vi "使用ActiveX讀取Excel檔案 to XY Graph.vi"() -> ()   [LabVIEW 2016]
panel:
  out "XY Graph":cluster{dbl[], dbl[]}(graph) caption="XY Graph - dark"
  out "Sheets":string[][](table)=[["", "土壤濕度"], ["11/24/2022 11:00", "40.7"], ["11/24/2022 11:30", "36.4"], ["11/24/2022 12:00", "36.4"], ["11/24/2022 12:30", "38.9"], ["11/24/2022 13:00", "38.3"], ["11/24/2022 13:30", "37.7"], ["11/24/2022 14:00", "36.9"], ["11/24/2022 14:30", "36.2"], ["11/24/2022 15:00", "35.4"], ["11/24/2022 15:30", "34.6"], ["11/24/2022 16:00", "33.8"], ["11/24/2022 16:30", "33.3"], ["11/24/2022 17:00", "32.7"], ["11/24/2022 17:30", "31.9"], ["11/24/2022 18:00", "31.3"], ["11/24/2022 18:30", "31"], ["11/24/2022 19:00", "30.5"], ["11/24/2022 19:30", "30.1"], ["11/24/2022 20:00", "29.8"], ["11/24/2022 20:30", "29.6"], ["11/24/2022 21:00", "29.4"], ["11/24/2022 21:30", "29.2"], ["11/24/2022 22:00", "29.1"], ["11/24/2022 22:30", "28.9"], ["11/24/2022 23:00", "28.8"], ["11/24/2022 23:30", "28.6"], ["11/25/2022 00:00", "28.5"], ["11/25/2022 00:30", "28.3"], ["11/25/2022 01:00", "28.3"], ["11/25/2022 01:30", "28.1"], ["11/25/2022 02:00", "28.1"], ["11/25/2022 02:30", "27.9"], ["11/25/2022 03:00", "27.9"], ["11/25/2022 03:30", "27.7"], ["11/25/2022 04:00", "27.7"], ["11/25/2022 04:30", "27.6"], ["11/25/2022 05:00", "27.5"], ["11/25/2022 05:30", "27.4"], ["11/25/2022 06:00", "27.4"], ["11/25/2022 06:30", "27.3"], ["11/25/2022 07:00", "27.3"], ["11/25/2022 07:30", "27.1"], ["11/25/2022 08:00", "27.1"], ["11/25/2022 08:30", "27.1"], ["11/25/2022 09:00", "27.1"], ["11/25/2022 09:30", "27.1"], ["11/25/2022 10:00", "27"], ["11/25/2022 10:30", "26.9"], ["11/25/2022 11:00", "26.9"], ["11/25/2022 11:30", "26.7"], ["11/25/2022 12:00", "26.6"], ["11/25/2022 12:30", "26.4"], ["11/25/2022 13:00", "26.3"], ["11/25/2022 13:30", "26.2"], ["11/25/2022 14:00", "26.1"], ["11/25/2022 14:30", "26"], ["11/25/2022 15:00", "25.9"], ["11/25/2022 15:30", "25.8"], ["11/25/2022 16:00", "25.7"], ["11/25/2022 16:30", "25.7"], ["11/25/2022 17:00", "25.7"], ["11/25/2022 17:30", "25.5"], ["11/25/2022 18:00", "25.4"], ["11/25/2022 18:30", "25.4"], ["11/25/2022 19:00", "25.4"], ["11/25/2022 19:30", "25.4"], ["11/25/2022 20:00", "25.4"], ["11/25/2022 20:30", "25.4"], ["11/25/2022 21:00", "25.3"], ["11/25/2022 21:30", "25.3"], ["11/25/2022 22:00", "25.2"], ["11/25/2022 22:30", "25.2"], ["11/25/2022 23:00", "25.2"], ["11/25/2022 23:30", "25.2"], ["11/26/2022 00:00", "25.2"], ["11/26/2022 00:30", "25.2"], ["11/26/2022 01:00", "25.2"], ["11/26/2022 01:30", "25.2"], ["11/26/2022 02:00", "25.2"], ["11/26/2022 02:30", "25"], ["11/26/2022 03:00", "25"], ["11/26/2022 03:30", "25.1"], ["11/26/2022 04:00", "25"], ["11/26/2022 04:30", "25"], ["11/26/2022 05:00", "25.1"], ["11/26/2022 05:30", "25"], ["11/26/2022 06:00", "25"], ["11/26/2022 06:30", "25.1"], ["11/26/2022 07:00", "25"], ["11/26/2022 07:30", "24.9"], ["11/26/2022 08:00", "25"], ["11/26/2022 08:30", "25"], ["11/26/2022 09:00", "25"], ["11/26/2022 09:30", "26.5"], ["11/26/2022 10:00", "27.7"], ["11/26/2022 10:30", "28"], ["11/26/2022 11:00", "27.9"], ["11/26/2022 11:30", "27.8"], ["11/26/2022 12:00", "27.6"], ["11/26/2022 12:30", "27.4"], ["11/26/2022 13:00", "27.1"], ["11/26/2022 13:30", "27.1"], ["11/26/2022 14:00", "26.9"], ["11/26/2022 14:30", "26.7"], ["11/26/2022 15:00", "26.5"], ["11/26/2022 15:30", "26.3"], ["11/26/2022 16:00", "26.3"], ["11/26/2022 16:30", "26.1"], ["11/26/2022 17:00", "26"], ["11/26/2022 17:30", "26"], ["11/26/2022 18:00", "26"], ["11/26/2022 18:30", "25.9"], ["11/26/2022 19:00", "25.8"], ["11/26/2022 19:30", "25.7"], ["11/26/2022 20:00", "25.7"], ["11/26/2022 20:30", "25.6"], ["11/26/2022 21:00", "25.6"], ["11/26/2022 21:30", "25.5"], ["11/26/2022 22:00", "25.5"], ["11/26/2022 22:30", "25.4"], ["11/26/2022 23:00", "25.4"], ["11/26/2022 23:30", "25.4"], ["11/27/2022 00:00", "25.4"], ["11/27/2022 00:30", "25.4"], ["11/27/2022 01:00", "25.4"], ["11/27/2022 01:30", "25.3"], ["11/27/2022 02:00", "25.3"], ["11/27/2022 02:30", "25.2"], ["11/27/2022 03:00", "25.2"], ["11/27/2022 03:30", "25.2"], ["11/27/2022 04:00", "25.2"], ["11/27/2022 04:30", "25.2"], ["11/27/2022 05:00", "25.2"], ["11/27/2022 05:30", "25.1"], ["11/27/2022 06:00", "25.1"], ["11/27/2022 06:30", "25"], ["11/27/2022 07:00", "25.1"], ["11/27/2022 07:30", "25"], ["11/27/2022 08:00", "25"], ["11/27/2022 08:30", "25"], ["11/27/2022 09:00", "25"], ["11/27/2022 09:30", "25"], ["11/27/2022 10:00", "25"], ["11/27/2022 10:30", "25.1"], ["11/27/2022 11:00", "25.1"], ["11/27/2022 11:30", "25.1"], ["11/27/2022 12:00", "25.1"], ["11/27/2022 12:30", "25"], ["11/27/2022 13:00", "25"], ["11/27/2022 13:30", "25"], ["11/27/2022 14:00", "25"], ["11/27/2022 14:30", "25"], ["11/27/2022 15:00", "25"], ["11/27/2022 15:30", "25"], ["11/27/2022 16:00", "24.9"], ["11/27/2022 16:30", "24.9"], ["11/27/2022 17:00", "25"], ["11/27/2022 17:30", "24.9"], ["11/27/2022 18:00", "24.9"], ["11/27/2022 18:30", "24.8"], ["11/27/2022 19:00", "24.9"], ["11/27/2022 19:30", "24.8"], ["11/27/2022 20:00", "24.8"], ["11/27/2022 20:30", "24.8"], ["11/27/2022 21:00", "24.8"], ["11/27/2022 21:30", "24.8"], ["11/27/2022 22:00", "24.6"], ["11/27/2022 22:30", "24.8"], ["11/27/2022 23:00", "24.7"], ["11/27/2022 23:30", "24.7"], ["11/28/2022 00:00", "24.6"], ["11/28/2022 00:30", "24.6"], ["11/28/2022 01:00", "24.6"], ["11/28/2022 01:30", "24.6"], ["11/28/2022 02:00", "24.6"], ["11/28/2022 02:30", "24.6"], ["11/28/2022 03:00", "24.6"], ["11/28/2022 03:30", "24.5"], ["11/28/2022 04:00", "24.5"], ["11/28/2022 04:30", "24.5"], ["11/28/2022 05:00", "24.5"], ["11/28/2022 05:30", "24.5"], ["11/28/2022 06:00", "24.5"], ["11/28/2022 06:30", "24.4"], ["11/28/2022 07:00", "24.4"], ["11/28/2022 07:30", "24.4"], ["11/28/2022 08:00", "24.4"], ["11/28/2022 08:30", "24.5"], ["11/28/2022 09:00", "24.4"], ["11/28/2022 09:30", "24.5"], ["11/28/2022 10:00", "24.5"], ["11/28/2022 10:30", "24.6"], ["11/28/2022 11:00", "24.6"], ["11/28/2022 11:30", "24.6"], ["11/28/2022 12:00", "24.7"], ["11/28/2022 12:30", "24.6"], ["11/28/2022 13:00", "24.6"], ["11/28/2022 13:30", "24.7"], ["11/28/2022 14:00", "24.8"], ["11/28/2022 14:30", "24.7"], ["11/28/2022 15:00", "24.7"], ["11/28/2022 15:30", "24.7"], ["11/28/2022 16:00", "24.8"], ["11/28/2022 16:30", "24.7"], ["11/28/2022 17:00", "24.7"], ["11/28/2022 17:30", "24.6"], ["11/28/2022 18:00", "24.6"], ["11/28/2022 18:30", "24.5"], ["11/28/2022 19:00", "24.6"], ["11/28/2022 19:30", "24.6"], ["11/28/2022 20:00", "24.5"], ["11/28/2022 20:30", "24.5"], ["11/28/2022 21:00", "24.5"], ["11/28/2022 21:30", "24.5"], ["11/28/2022 22:00", "24.5"], ["11/28/2022 22:30", "24.3"], ["11/28/2022 23:00", "24.4"], ["11/28/2022 23:30", "24.4"], ["11/29/2022 00:00", "24.3"], ["11/29/2022 00:30", "24.3"], ["11/29/2022 01:00", "24.3"], ["11/29/2022 01:30", "24.3"], ["11/29/2022 02:00", "24.3"], ["11/29/2022 02:30", "24.3"], ["11/29/2022 03:00", "24.3"], ["11/29/2022 03:30", "24.3"], ["11/29/2022 04:00", "24.3"], ["11/29/2022 04:30", "24.3"], ["11/29/2022 05:00", "24.3"], ["11/29/2022 05:30", "24.2"], ["11/29/2022 06:00", "24.1"], ["11/29/2022 06:30", "24.2"], ["11/29/2022 07:00", "24.1"], ["11/29/2022 07:30", "24.2"], ["11/29/2022 08:00", "24.2"], ["11/29/2022 08:30", "24.1"], ["11/29/2022 09:00", "24.2"], ["11/29/2022 09:30", "24.1"], ["11/29/2022 10:00", "24.3"], ["11/29/2022 10:30", "24.3"], ["11/29/2022 11:00", "24.4"], ["11/29/2022 11:30", "24.4"], ["11/29/2022 12:00", "24.4"], ["11/29/2022 12:30", "24.5"], ["11/29/2022 13:00", "24.3"], ["11/29/2022 13:30", "24.5"], ["11/29/2022 14:00", "24.6"], ["11/29/2022 14:30", "24.6"], ["11/29/2022 15:00", "24.5"], ["11/29/2022 15:30", "24.5"], ["11/29/2022 16:00", "24.6"], ["11/29/2022 16:30", "24.6"], ["11/29/2022 17:00", "24.6"], ["11/29/2022 17:30", "24.6"], ["11/29/2022 18:00", "24.5"], ["11/29/2022 18:30", "24.5"], ["11/29/2022 19:00", "24.5"], ["11/29/2022 19:30", "24.4"], ["11/29/2022 20:00", "24.4"], ["11/29/2022 20:30", "24.5"], ["11/29/2022 21:00", "24.5"], ["11/29/2022 21:30", "24.4"], ["11/29/2022 22:00", "24.3"], ["11/29/2022 22:30", "24.3"], ["11/29/2022 23:00", "24.3"], ["11/29/2022 23:30", "24.3"], ["11/30/2022 00:00", "24.3"], ["11/30/2022 00:30", "24.3"], ["11/30/2022 01:00", "24.3"], ["11/30/2022 01:30", "24.3"], ["11/30/2022 02:00", "24.3"], ["11/30/2022 02:30", "24.2"], ["11/30/2022 03:00", "24.2"], ["11/30/2022 03:30", "24.2"], ["11/30/2022 04:00", "24.2"], ["11/30/2022 04:30", "24.1"], ["11/30/2022 05:00", "24.1"], ["11/30/2022 05:30", "24.1"], ["11/30/2022 06:00", "24.1"], ["11/30/2022 06:30", "24.1"], ["11/30/2022 07:00", "24.1"], ["11/30/2022 07:30", "24.1"], ["11/30/2022 08:00", "24.1"], ["11/30/2022 08:30", "24.1"], ["11/30/2022 09:00", "24.1"], ["11/30/2022 09:30", "24.1"], ["11/30/2022 10:00", "24.3"], ["11/30/2022 10:30", "24.3"], ["11/30/2022 11:00", "24.3"], ["11/30/2022 11:30", "24.3"], ["11/30/2022 12:00", "24.4"], ["11/30/2022 12:30", "24.3"], ["11/30/2022 13:00", "24.3"], ["11/30/2022 13:30", "24.3"], ["11/30/2022 14:00", "24.4"], ["11/30/2022 14:30", "24.4"], ["11/30/2022 15:00", "24.5"], ["11/30/2022 15:30", "24.4"], ["11/30/2022 16:00", "24.3"], ["11/30/2022 16:30", "24.4"], ["11/30/2022 17:00", "24.3"], ["11/30/2022 17:30", "24.3"], ["11/30/2022 18:00", "24.3"], ["11/30/2022 18:30", "24.3"], ["11/30/2022 19:00", "24.3"], ["11/30/2022 19:30", "24.2"], ["11/30/2022 20:00", "24.2"], ["11/30/2022 20:30", "24.1"], ["11/30/2022 21:00", "24.1"], ["11/30/2022 21:30", "24.2"], ["11/30/2022 22:00", "24.1"], ["11/30/2022 22:30", "24.1"], ["11/30/2022 23:00", "24.1"], ["11/30/2022 23:30", "24.1"], ["12/01/2022 00:00", "23.9"], ["12/01/2022 00:30", "24"], ["12/01/2022 01:00", "24.1"], ["12/01/2022 01:30", "24"], ["12/01/2022 02:00", "23.9"], ["12/01/2022 02:30", "23.9"], ["12/01/2022 03:00", "23.9"], ["12/01/2022 03:30", "23.9"], ["12/01/2022 04:00", "23.9"], ["12/01/2022 04:30", "23.9"], ["12/01/2022 05:00", "23.7"], ["12/01/2022 05:30", "23.8"], ["12/01/2022 06:00", "23.8"], ["12/01/2022 06:30", "23.7"], ["12/01/2022 07:00", "23.7"], ["12/01/2022 07:30", "23.7"], ["12/01/2022 08:00", "23.7"], ["12/01/2022 08:30", "23.7"], ["12/01/2022 09:00", "23.7"], ["12/01/2022 09:30", "23.9"], ["12/01/2022 10:00", "23.9"], ["12/01/2022 10:30", "24"], ["12/01/2022 11:00", "24"], ["12/01/2022 11:30", "24.1"], ["12/01/2022 12:00", "24.1"], ["12/01/2022 12:30", "24.1"], ["12/01/2022 13:00", "24.1"], ["12/01/2022 13:30", "24.1"], ["12/01/2022 14:00", "24.2"], ["12/01/2022 14:30", "24.1"], ["12/01/2022 15:00", "24.1"], ["12/01/2022 15:30", "24.2"], ["12/01/2022 16:00", "24.3"], ["12/01/2022 16:30", "24.2"], ["12/01/2022 17:00", "24.2"], ["12/01/2022 17:30", "24.1"], ["12/01/2022 18:00", "24.1"], ["12/01/2022 18:30", "24.1"], ["12/01/2022 19:00", "24.1"], ["12/01/2022 19:30", "24.1"], ["12/01/2022 20:00", "24.1"], ["12/01/2022 20:30", "24"], ["12/01/2022 21:00", "24.1"], ["12/01/2022 21:30", "24"], ["12/01/2022 22:00", "24"], ["12/01/2022 22:30", "23.9"], ["12/01/2022 23:00", "23.8"], ["12/01/2022 23:30", "23.8"], ["12/02/2022 00:00", "23.7"], ["12/02/2022 00:30", "23.8"], ["12/02/2022 01:00", "23.8"], ["12/02/2022 01:30", "23.7"], ["12/02/2022 02:00", "23.8"], ["12/02/2022 02:30", "23.8"], ["12/02/2022 03:00", "23.7"], ["12/02/2022 03:30", "23.7"], ["12/02/2022 04:00", "23.7"], ["12/02/2022 04:30", "23.7"], ["12/02/2022 05:00", "23.7"], ["12/02/2022 05:30", "23.7"], ["12/02/2022 06:00", "23.7"], ["12/02/2022 06:30", "23.7"], ["12/02/2022 07:00", "23.7"], ["12/02/2022 07:30", "23.7"], ["12/02/2022 08:00", "23.7"], ["12/02/2022 08:30", "23.7"], ["12/02/2022 09:00", "23.7"], ["12/02/2022 09:30", "24.1"], ["12/02/2022 10:00", "24.1"], ["12/02/2022 10:30", "24.1"], ["12/02/2022 11:00", "24.1"], ["12/02/2022 11:30", "24.1"], ["12/02/2022 12:00", "24.1"], ["12/02/2022 12:30", "24.1"], ["12/02/2022 13:00", "24.1"], ["12/02/2022 13:30", "24.1"], ["12/02/2022 14:00", "24.3"], ["12/02/2022 14:30", "24.3"], ["12/02/2022 15:00", "24.1"], ["12/02/2022 15:30", "24.1"], ["12/02/2022 16:00", "24.1"], ["12/02/2022 16:30", "24.2"], ["12/02/2022 17:00", "24.1"], ["12/02/2022 17:30", "23.8"], ["12/02/2022 18:00", "24.1"], ["12/02/2022 18:30", "24.1"], ["12/02/2022 19:00", "24.1"], ["12/02/2022 19:30", "24"], ["12/02/2022 20:00", "24.1"], ["12/02/2022 20:30", "23.9"], ["12/02/2022 21:00", "23.9"], ["12/02/2022 21:30", "23.9"], ["12/02/2022 22:00", "23.9"], ["12/02/2022 22:30", "23.9"], ["12/02/2022 23:00", "23.9"], ["12/02/2022 23:30", "23.7"], ["12/03/2022 00:00", "23.7"], ["12/03/2022 00:30", "23.8"], ["12/03/2022 01:00", "23.7"], ["12/03/2022 01:30", "23.7"], ["12/03/2022 02:00", "23.7"], ["12/03/2022 02:30", "23.7"], ["12/03/2022 03:00", "23.7"], ["12/03/2022 03:30", "23.6"], ["12/03/2022 04:00", "23.6"], ["12/03/2022 04:30", "23.5"], ["12/03/2022 05:00", "23.5"], ["12/03/2022 05:30", "23.5"], ["12/03/2022 06:00", "23.7"], ["12/03/2022 06:30", "23.6"], ["12/03/2022 07:00", "23.5"], ["12/03/2022 07:30", "23.5"], ["12/03/2022 08:00", "23.5"], ["12/03/2022 08:30", "23.5"], ["12/03/2022 09:00", "23.6"], ["12/03/2022 09:30", "23.7"], ["12/03/2022 10:00", "23.7"], ["12/03/2022 10:30", "23.8"], ["12/03/2022 11:00", "23.9"], ["12/03/2022 11:30", "23.9"], ["12/03/2022 12:00", "24"], ["12/03/2022 12:30", "24"], ["12/03/2022 13:00", "24"], ["12/03/2022 13:30", "23.9"], ["12/03/2022 14:00", "24.1"], ["12/03/2022 14:30", "24.1"], ["12/03/2022 15:00", "24.1"], ["12/03/2022 15:30", "24.1"], ["12/03/2022 16:00", "24.1"], ["12/03/2022 16:30", "24.1"], ["12/03/2022 17:00", "24.1"], ["12/03/2022 17:30", "24.1"], ["12/03/2022 18:00", "23.9"], ["12/03/2022 18:30", "24"], ["12/03/2022 19:00", "23.9"], ["12/03/2022 19:30", "23.9"], ["12/03/2022 20:00", "23.9"], ["12/03/2022 20:30", "23.9"], ["12/03/2022 21:00", "23.9"], ["12/03/2022 21:30", "23.7"], ["12/03/2022 22:00", "23.7"], ["12/03/2022 22:30", "23.7"], ["12/03/2022 23:00", "23.7"], ["12/03/2022 23:30", "23.7"], ["12/04/2022 00:00", "23.7"], ["12/04/2022 00:30", "23.7"], ["12/04/2022 01:00", "23.7"], ["12/04/2022 01:30", "23.7"], ["12/04/2022 02:00", "23.7"], ["12/04/2022 02:30", "23.7"], ["12/04/2022 03:00", "23.6"], ["12/04/2022 03:30", "23.5"], ["12/04/2022 04:00", "23.7"], ["12/04/2022 04:30", "23.6"], ["12/04/2022 05:00", "23.6"], ["12/04/2022 05:30", "23.6"], ["12/04/2022 06:00", "23.6"], ["12/04/2022 06:30", "23.6"], ["12/04/2022 07:00", "23.6"], ["12/04/2022 07:30", "23.5"], ["12/04/2022 08:00", "23.6"], ["12/04/2022 08:30", "23.5"], ["12/04/2022 09:00", "23.6"], ["12/04/2022 09:30", "23.7"], ["12/04/2022 10:00", "23.7"], ["12/04/2022 10:30", "23.7"], ["12/04/2022 11:00", "23.7"], ["12/04/2022 11:30", "23.7"], ["12/04/2022 12:00", "23.7"], ["12/04/2022 12:30", "23.8"], ["12/04/2022 13:00", "23.9"], ["12/04/2022 13:30", "23.9"], ["12/04/2022 14:00", "24"], ["12/04/2022 14:30", "23.9"], ["12/04/2022 15:00", "24.1"], ["12/04/2022 15:30", "24.1"], ["12/04/2022 16:00", "24.1"], ["12/04/2022 16:30", "24.1"], ["12/04/2022 17:00", "24.1"], ["12/04/2022 17:30", "23.9"], ["12/04/2022 18:00", "23.9"], ["12/04/2022 18:30", "23.9"], ["12/04/2022 19:00", "23.9"], ["12/04/2022 19:30", "23.7"], ["12/04/2022 20:00", "23.7"], ["12/04/2022 20:30", "23.7"], ["12/04/2022 21:00", "23.7"], ["12/04/2022 21:30", "23.7"], ["12/04/2022 22:00", "23.7"], ["12/04/2022 22:30", "23.7"], ["12/04/2022 23:00", "23.7"], ["12/04/2022 23:30", "23.7"], ["12/05/2022 00:00", "23.7"], ["12/05/2022 00:30", "23.7"], ["12/05/2022 01:00", "23.7"], ["12/05/2022 01:30", "23.7"], ["12/05/2022 02:00", "23.6"], ["12/05/2022 02:30", "23.5"], ["12/05/2022 03:00", "23.6"], ["12/05/2022 03:30", "23.6"], ["12/05/2022 04:00", "23.5"], ["12/05/2022 04:30", "23.5"], ["12/05/2022 05:00", "23.5"], ["12/05/2022 05:30", "23.5"], ["12/05/2022 06:00", "23.5"], ["12/05/2022 06:30", "23.5"], ["12/05/2022 07:00", "23.5"], ["12/05/2022 07:30", "23.5"], ["12/05/2022 08:00", "23.5"], ["12/05/2022 08:30", "23.5"], ["12/05/2022 09:00", "23.5"], ["12/05/2022 09:30", "23.6"], ["12/05/2022 10:00", "23.6"], ["12/05/2022 10:30", "23.7"], ["12/05/2022 11:00", "23.7"], ["12/05/2022 11:30", "23.9"], ["12/05/2022 12:00", "23.7"], ["12/05/2022 12:30", "23.7"], ["12/05/2022 13:00", "23.7"], ["12/05/2022 13:30", "23.9"], ["12/05/2022 14:00", "23.9"], ["12/05/2022 14:30", "23.8"], ["12/05/2022 15:00", "23.9"], ["12/05/2022 15:30", "23.8"], ["12/05/2022 16:00", "23.9"], ["12/05/2022 16:30", "23.9"], ["12/05/2022 17:00", "23.7"], ["12/05/2022 17:30", "23.8"], ["12/05/2022 18:00", "23.8"], ["12/05/2022 18:30", "23.7"], ["12/05/2022 19:00", "23.7"], ["12/05/2022 19:30", "23.7"], ["12/05/2022 20:00", "23.7"], ["12/05/2022 20:30", "23.6"], ["12/05/2022 21:00", "23.7"], ["12/05/2022 21:30", "23.5"], ["12/05/2022 22:00", "23.5"], ["12/05/2022 22:30", "23.5"], ["12/05/2022 23:00", "23.5"], ["12/05/2022 23:30", "23.5"], ["12/06/2022 00:00", "23.5"], ["12/06/2022 00:30", "23.5"], ["12/06/2022 01:00", "23.4"], ["12/06/2022 01:30", "23.5"], ["12/06/2022 02:00", "23.5"], ["12/06/2022 02:30", "23.5"], ["12/06/2022 03:00", "23.5"], ["12/06/2022 03:30", "23.4"], ["12/06/2022 04:00", "23.3"], ["12/06/2022 04:30", "23.4"], ["12/06/2022 05:00", "23.3"], ["12/06/2022 05:30", "23.3"], ["12/06/2022 06:00", "23.3"], ["12/06/2022 06:30", "23.3"], ["12/06/2022 07:00", "23.3"], ["12/06/2022 07:30", "23.3"], ["12/06/2022 08:00", "23.3"], ["12/06/2022 08:30", "23.3"], ["12/06/2022 09:00", "23.3"], ["12/06/2022 09:30", "23.3"], ["12/06/2022 10:00", "23.3"], ["12/06/2022 10:30", "23.4"], ["12/06/2022 11:00", "23.4"], ["12/06/2022 11:30", "23.5"], ["12/06/2022 12:00", "23.5"], ["12/06/2022 12:30", "23.5"], ["12/06/2022 13:00", "23.5"], ["12/06/2022 13:30", "23.6"], ["12/06/2022 14:00", "23.6"], ["12/06/2022 14:30", "23.6"], ["12/06/2022 15:00", "23.7"], ["12/06/2022 15:30", "23.7"], ["12/06/2022 16:00", "23.7"], ["12/06/2022 16:30", "23.5"], ["12/06/2022 17:00", "23.5"], ["12/06/2022 17:30", "23.4"], ["12/06/2022 18:00", "23.5"], ["12/06/2022 18:30", "23.5"], ["12/06/2022 19:00", "23.5"], ["12/06/2022 19:30", "23.4"], ["12/06/2022 20:00", "23.4"], ["12/06/2022 20:30", "23.3"], ["12/06/2022 21:00", "23.4"], ["12/06/2022 21:30", "23.3"], ["12/06/2022 22:00", "23.4"], ["12/06/2022 22:30", "23.3"], ["12/06/2022 23:00", "23.4"], ["12/06/2022 23:30", "23.3"], ["12/07/2022 00:00", "23.4"], ["12/07/2022 00:30", "23.3"], ["12/07/2022 01:00", "23.4"], ["12/07/2022 01:30", "23.3"], ["12/07/2022 02:00", "23.3"], ["12/07/2022 02:30", "23.3"], ["12/07/2022 03:00", "23.3"], ["12/07/2022 03:30", "23.3"], ["12/07/2022 04:00", "23.3"], ["12/07/2022 04:30", "23.3"], ["12/07/2022 05:00", "23.3"], ["12/07/2022 05:30", "23.3"], ["12/07/2022 06:00", "23.3"], ["12/07/2022 06:30", "23.3"], ["12/07/2022 07:00", "23.3"], ["12/07/2022 07:30", "23.3"], ["12/07/2022 08:00", "23.3"], ["12/07/2022 08:30", "23.3"], ["12/07/2022 09:00", "23.3"], ["12/07/2022 09:30", "23.3"], ["12/07/2022 10:00", "23.3"], ["12/07/2022 10:30", "23.5"], ["12/07/2022 11:00", "23.5"], ["12/07/2022 11:30", "23.5"], ["12/07/2022 12:00", "23.5"], ["12/07/2022 12:30", "23.5"], ["12/07/2022 13:00", "23.5"], ["12/07/2022 13:30", "23.5"], ["12/07/2022 14:00", "23.6"], ["12/07/2022 14:30", "23.5"], ["12/07/2022 15:00", "23.5"], ["12/07/2022 15:30", "23.5"], ["12/07/2022 16:00", "23.5"], ["12/07/2022 16:30", "23.5"], ["12/07/2022 17:00", "23.5"], ["12/07/2022 17:30", "23.5"], ["12/07/2022 18:00", "23.5"], ["12/07/2022 18:30", "23.5"], ["12/07/2022 19:00", "23.5"], ["12/07/2022 19:30", "23.5"], ["12/07/2022 20:00", "23.4"], ["12/07/2022 20:30", "23.4"], ["12/07/2022 21:00", "23.4"], ["12/07/2022 21:30", "23.3"], ["12/07/2022 22:00", "23.3"], ["12/07/2022 22:30", "23.4"], ["12/07/2022 23:00", "23.3"], ["12/07/2022 23:30", "23.3"], ["12/08/2022 00:00", "23.3"], ["12/08/2022 00:30", "23.3"], ["12/08/2022 01:00", "23.3"], ["12/08/2022 01:30", "23.2"], ["12/08/2022 02:00", "23.3"], ["12/08/2022 02:30", "23.2"], ["12/08/2022 03:00", "23.2"], ["12/08/2022 03:30", "23.1"], ["12/08/2022 04:00", "23.2"], ["12/08/2022 04:30", "23.2"], ["12/08/2022 05:00", "23.2"], ["12/08/2022 05:30", "23.2"], ["12/08/2022 06:00", "23.1"], ["12/08/2022 06:30", "23.2"], ["12/08/2022 07:00", "23.1"], ["12/08/2022 07:30", "23.1"], ["12/08/2022 08:00", "23"], ["12/08/2022 08:30", "23.1"], ["12/08/2022 09:00", "23"], ["12/08/2022 09:30", "23.1"], ["12/08/2022 10:00", "23.1"], ["12/08/2022 10:30", "23.2"], ["12/08/2022 11:00", "23.2"], ["12/08/2022 11:30", "23.3"], ["12/08/2022 12:00", "23.3"], ["12/08/2022 12:30", "23.4"], ["12/08/2022 13:00", "23.4"], ["12/08/2022 13:30", "23.4"], ["12/08/2022 14:00", "23.5"], ["12/08/2022 14:30", "23.5"], ["12/08/2022 15:00", "23.5"], ["12/08/2022 15:30", "23.5"], ["12/08/2022 16:00", "23.5"], ["12/08/2022 16:30", "23.3"], ["12/08/2022 17:00", "23.4"], ["12/08/2022 17:30", "23.5"], ["12/08/2022 18:00", "23.4"], ["12/08/2022 18:30", "23.5"], ["12/08/2022 19:00", "23.5"], ["12/08/2022 19:30", "23.5"], ["12/08/2022 20:00", "23.5"], ["12/08/2022 20:30", "23.4"], ["12/08/2022 21:00", "23.4"], ["12/08/2022 21:30", "23.3"], ["12/08/2022 22:00", "23.3"], ["12/08/2022 22:30", "23.3"], ["12/08/2022 23:00", "23.3"], ["12/08/2022 23:30", "23.2"], ["12/09/2022 00:00", "23.2"], ["12/09/2022 00:30", "23.2"], ["12/09/2022 01:00", "23.2"], ["12/09/2022 01:30", "23.2"], ["12/09/2022 02:00", "23.2"], ["12/09/2022 02:30", "23.2"], ["12/09/2022 03:00", "23.2"], ["12/09/2022 03:30", "23.1"], ["12/09/2022 04:00", "23"], ["12/09/2022 04:30", "23.1"], ["12/09/2022 05:00", "23"], ["12/09/2022 05:30", "23.1"], ["12/09/2022 06:00", "22.9"], ["12/09/2022 06:30", "22.9"], ["12/09/2022 07:00", "23"], ["12/09/2022 07:30", "23"], ["12/09/2022 08:00", "22.9"], ["12/09/2022 08:30", "22.9"], ["12/09/2022 09:00", "22.9"], ["12/09/2022 09:30", "22.8"], ["12/09/2022 10:00", "22.9"], ["12/09/2022 10:30", "22.9"], ["12/09/2022 11:00", "23.1"], ["12/09/2022 11:30", "23.2"], ["12/09/2022 12:00", "23.2"], ["12/09/2022 12:30", "23.1"], ["12/09/2022 13:00", "23.2"], ["12/09/2022 13:30", "23.3"], ["12/09/2022 14:00", "23.3"], ["12/09/2022 14:30", "23.3"], ["12/09/2022 15:00", "23.3"], ["12/09/2022 15:30", "23.3"], ["12/09/2022 16:00", "23.2"], ["12/09/2022 16:30", "23.3"], ["12/09/2022 17:00", "23.2"], ["12/09/2022 17:30", "23.2"], ["12/09/2022 18:00", "23.2"], ["12/09/2022 18:30", "23.2"], ["12/09/2022 19:00", "23.2"], ["12/09/2022 19:30", "23.2"], ["12/09/2022 20:00", "23.1"], ["12/09/2022 20:30", "23.1"], ["12/09/2022 21:00", "23.1"], ["12/09/2022 21:30", "23"], ["12/09/2022 22:00", "23.2"], ["12/09/2022 22:30", "23.2"], ["12/09/2022 23:00", "22.9"], ["12/09/2022 23:30", "23"], ["12/10/2022 00:00", "23.1"], ["12/10/2022 00:30", "23.1"], ["12/10/2022 01:00", "23"], ["12/10/2022 01:30", "22.9"], ["12/10/2022 02:00", "22.9"], ["12/10/2022 02:30", "22.9"], ["12/10/2022 03:00", "23.1"], ["12/10/2022 03:30", "22.9"], ["12/10/2022 04:00", "22.9"], ["12/10/2022 04:30", "22.9"], ["12/10/2022 05:00", "22.9"], ["12/10/2022 05:30", "22.9"], ["12/10/2022 06:00", "22.9"], ["12/10/2022 06:30", "22.9"], ["12/10/2022 07:00", "22.9"], ["12/10/2022 07:30", "22.9"], ["12/10/2022 08:00", "22.9"], ["12/10/2022 08:30", "22.9"], ["12/10/2022 09:00", "22.8"], ["12/10/2022 09:30", "22.9"], ["12/10/2022 10:00", "23.7"], ["12/10/2022 10:30", "24.3"], ["12/10/2022 11:00", "24.5"], ["12/10/2022 11:30", "24.6"], ["12/10/2022 12:00", "24.8"], ["12/10/2022 12:30", "24.8"], ["12/10/2022 13:00", "24.9"], ["12/10/2022 13:30", "24.9"], ["12/10/2022 14:00", "24.8"], ["12/10/2022 14:30", "24.8"], ["12/10/2022 15:00", "24.7"], ["12/10/2022 15:30", "24.7"], ["12/10/2022 16:00", "24.6"], ["12/10/2022 16:30", "24.6"], ["12/10/2022 17:00", "24.6"], ["12/10/2022 17:30", "24.5"], ["12/10/2022 18:00", "24.5"], ["12/10/2022 18:30", "24.5"], ["12/10/2022 19:00", "24.3"], ["12/10/2022 19:30", "24.4"], ["12/10/2022 20:00", "24.4"], ["12/10/2022 20:30", "24.3"], ["12/10/2022 21:00", "24.3"], ["12/10/2022 21:30", "24.3"], ["12/10/2022 22:00", "24.3"], ["12/10/2022 22:30", "24.2"], ["12/10/2022 23:00", "24.2"], ["12/10/2022 23:30", "24.2"], ["12/11/2022 00:00", "24.1"], ["12/11/2022 00:30", "24.1"], ["12/11/2022 01:00", "24"], ["12/11/2022 01:30", "24"], ["12/11/2022 02:00", "24"], ["12/11/2022 02:30", "24"], ["12/11/2022 03:00", "23.9"], ["12/11/2022 03:30", "23.8"], ["12/11/2022 04:00", "23.8"], ["12/11/2022 04:30", "23.7"], ["12/11/2022 05:00", "23.7"], ["12/11/2022 05:30", "23.7"], ["12/11/2022 06:00", "23.7"], ["12/11/2022 06:30", "23.7"], ["12/11/2022 07:00", "23.5"], ["12/11/2022 07:30", "23.6"], ["12/11/2022 08:00", "23.6"], ["12/11/2022 08:30", "23.5"], ["12/11/2022 09:00", "23.5"], ["12/11/2022 09:30", "23.5"], ["12/11/2022 10:00", "23.6"], ["12/11/2022 10:30", "23.5"], ["12/11/2022 11:00", "23.5"], ["12/11/2022 11:30", "23.6"], ["12/11/2022 12:00", "23.5"], ["12/11/2022 12:30", "23.5"], ["12/11/2022 13:00", "23.5"], ["12/11/2022 13:30", "23.5"], ["12/11/2022 14:00", "23.5"], ["12/11/2022 14:30", "23.5"], ["12/11/2022 15:00", "23.5"], ["12/11/2022 15:30", "23.5"], ["12/11/2022 16:00", "23.5"], ["12/11/2022 16:30", "23.5"], ["12/11/2022 17:00", "23.5"], ["12/11/2022 17:30", "23.5"], ["12/11/2022 18:00", "23.4"], ["12/11/2022 18:30", "23.5"], ["12/11/2022 19:00", "23.3"], ["12/11/2022 19:30", "23.5"], ["12/11/2022 20:00", "23.4"], ["12/11/2022 20:30", "23.3"], ["12/11/2022 21:00", "23.3"], ["12/11/2022 21:30", "23.4"], ["12/11/2022 22:00", "23.3"], ["12/11/2022 22:30", "23.3"], ["12/11/2022 23:00", "23.3"], ["12/11/2022 23:30", "23.2"], ["12/12/2022 00:00", "23.3"], ["12/12/2022 00:30", "23.3"], ["12/12/2022 01:00", "23.2"], ["12/12/2022 01:30", "23.2"], ["12/12/2022 02:00", "23.2"], ["12/12/2022 02:30", "23.1"], ["12/12/2022 03:00", "23.2"], ["12/12/2022 03:30", "23.1"], ["12/12/2022 04:00", "23.1"], ["12/12/2022 04:30", "23.1"], ["12/12/2022 05:00", "23.1"], ["12/12/2022 05:30", "23"], ["12/12/2022 06:00", "22.9"], ["12/12/2022 06:30", "23.1"], ["12/12/2022 07:00", "22.9"], ["12/12/2022 07:30", "22.9"], ["12/12/2022 08:00", "22.9"], ["12/12/2022 08:30", "22.9"], ["12/12/2022 09:00", "23"], ["12/12/2022 09:30", "22.9"], ["12/12/2022 10:00", "22.9"], ["12/12/2022 10:30", "22.9"], ["12/12/2022 11:00", "23.1"], ["12/12/2022 11:30", "23.1"], ["12/12/2022 12:00", "23.1"], ["12/12/2022 12:30", "23"], ["12/12/2022 13:00", "23.1"], ["12/12/2022 13:30", "23.1"], ["12/12/2022 14:00", "23.2"], ["12/12/2022 14:30", "23.1"], ["12/12/2022 15:00", "23.3"], ["12/12/2022 15:30", "23.2"], ["12/12/2022 16:00", "23.1"], ["12/12/2022 16:30", "23.1"], ["12/12/2022 17:00", "23.1"], ["12/12/2022 17:30", "23.1"], ["12/12/2022 18:00", "23"], ["12/12/2022 18:30", "22.9"], ["12/12/2022 19:00", "22.9"], ["12/12/2022 19:30", "23"], ["12/12/2022 20:00", "22.9"], ["12/12/2022 20:30", "22.9"], ["12/12/2022 21:00", "22.9"], ["12/12/2022 21:30", "22.9"], ["12/12/2022 22:00", "22.9"], ["12/12/2022 22:30", "22.9"], ["12/12/2022 23:00", "22.9"], ["12/12/2022 23:30", "22.9"], ["12/13/2022 00:00", "22.9"], ["12/13/2022 00:30", "22.9"], ["12/13/2022 01:00", "22.8"], ["12/13/2022 01:30", "22.9"], ["12/13/2022 02:00", "22.8"], ["12/13/2022 02:30", "22.8"], ["12/13/2022 03:00", "22.8"], ["12/13/2022 03:30", "22.7"], ["12/13/2022 04:00", "22.7"], ["12/13/2022 04:30", "22.8"], ["12/13/2022 05:00", "22.7"], ["12/13/2022 05:30", "22.7"], ["12/13/2022 06:00", "22.7"], ["12/13/2022 06:30", "22.7"], ["12/13/2022 07:00", "22.7"], ["12/13/2022 07:30", "22.7"], ["12/13/2022 08:00", "22.7"], ["12/13/2022 08:30", "22.7"], ["12/13/2022 09:00", "22.7"], ["12/13/2022 09:30", "22.7"], ["12/13/2022 10:00", "22.8"], ["12/13/2022 10:30", "22.8"], ["12/13/2022 11:00", "22.9"], ["12/13/2022 11:30", "22.9"], ["12/13/2022 12:00", "22.9"], ["12/13/2022 12:30", "22.9"], ["12/13/2022 13:00", "22.9"], ["12/13/2022 13:30", "22.9"], ["12/13/2022 14:00", "22.9"], ["12/13/2022 14:30", "23.1"], ["12/13/2022 15:00", "23.1"], ["12/13/2022 15:30", "23.1"], ["12/13/2022 16:00", "23"], ["12/13/2022 16:30", "23.1"], ["12/13/2022 17:00", "22.9"], ["12/13/2022 17:30", "22.9"], ["12/13/2022 18:00", "23.1"], ["12/13/2022 18:30", "23.1"], ["12/13/2022 19:00", "22.9"], ["12/13/2022 19:30", "22.9"], ["12/13/2022 20:00", "22.9"], ["12/13/2022 20:30", "22.8"], ["12/13/2022 21:00", "22.9"], ["12/13/2022 21:30", "22.8"], ["12/13/2022 22:00", "22.8"], ["12/13/2022 22:30", "22.8"], ["12/13/2022 23:00", "22.8"], ["12/13/2022 23:30", "22.7"], ["12/14/2022 00:00", "22.7"], ["12/14/2022 00:30", "22.7"], ["12/14/2022 01:00", "22.7"], ["12/14/2022 01:30", "22.7"], ["12/14/2022 02:00", "22.7"], ["12/14/2022 02:30", "22.7"], ["12/14/2022 03:00", "22.7"], ["12/14/2022 03:30", "22.7"], ["12/14/2022 04:00", "22.7"], ["12/14/2022 04:30", "22.7"], ["12/14/2022 05:00", "22.7"], ["12/14/2022 05:30", "22.6"], ["12/14/2022 06:00", "22.6"], ["12/14/2022 06:30", "22.6"], ["12/14/2022 07:00", "22.6"], ["12/14/2022 07:30", "22.7"], ["12/14/2022 08:00", "22.6"], ["12/14/2022 08:30", "22.5"], ["12/14/2022 09:00", "22.6"], ["12/14/2022 09:30", "22.7"], ["12/14/2022 10:00", "22.5"], ["12/14/2022 10:30", "22.7"], ["12/14/2022 11:00", "22.7"], ["12/14/2022 11:30", "22.7"], ["12/14/2022 12:00", "22.7"], ["12/14/2022 12:30", "22.7"], ["12/14/2022 13:00", "22.7"], ["12/14/2022 13:30", "22.7"], ["12/14/2022 14:00", "22.7"], ["12/14/2022 14:30", "22.8"], ["12/14/2022 15:00", "22.8"], ["12/14/2022 15:30", "22.7"], ["12/14/2022 16:00", "22.7"], ["12/14/2022 16:30", "22.7"], ["12/14/2022 17:00", "22.7"], ["12/14/2022 17:30", "22.8"], ["12/14/2022 18:00", "22.8"], ["12/14/2022 18:30", "22.7"], ["12/14/2022 19:00", "22.7"], ["12/14/2022 19:30", "22.8"], ["12/14/2022 20:00", "22.7"], ["12/14/2022 20:30", "22.7"], ["12/14/2022 21:00", "22.7"], ["12/14/2022 21:30", "22.7"], ["12/14/2022 22:00", "22.7"], ["12/14/2022 22:30", "22.7"], ["12/14/2022 23:00", "22.7"], ["12/14/2022 23:30", "22.7"], ["12/15/2022 00:00", "22.7"], ["12/15/2022 00:30", "22.6"], ["12/15/2022 01:00", "22.7"], ["12/15/2022 01:30", "22.7"], ["12/15/2022 02:00", "22.7"], ["12/15/2022 02:30", "22.6"], ["12/15/2022 03:00", "22.6"], ["12/15/2022 03:30", "22.7"], ["12/15/2022 04:00", "22.6"], ["12/15/2022 04:30", "22.6"], ["12/15/2022 05:00", "22.5"], ["12/15/2022 05:30", "22.6"], ["12/15/2022 06:00", "22.6"], ["12/15/2022 06:30", "22.6"], ["12/15/2022 07:00", "22.6"], ["12/15/2022 07:30", "22.6"], ["12/15/2022 08:00", "22.5"], ["12/15/2022 08:30", "22.6"], ["12/15/2022 09:00", "22.5"], ["12/15/2022 09:30", "22.5"], ["12/15/2022 10:00", "22.7"], ["12/15/2022 10:30", "22.7"], ["12/15/2022 11:00", "22.7"], ["12/15/2022 11:30", "22.7"], ["12/15/2022 12:00", "22.8"], ["12/15/2022 12:30", "22.8"], ["12/15/2022 13:00", "22.7"], ["12/15/2022 13:30", "22.9"], ["12/15/2022 14:00", "22.8"], ["12/15/2022 14:30", "22.9"], ["12/15/2022 15:00", "22.9"], ["12/15/2022 15:30", "22.8"], ["12/15/2022 16:00", "22.9"], ["12/15/2022 16:30", "22.9"], ["12/15/2022 17:00", "22.9"], ["12/15/2022 17:30", "22.7"], ["12/15/2022 18:00", "22.9"], ["12/15/2022 18:30", "22.9"], ["12/15/2022 19:00", "22.8"], ["12/15/2022 19:30", "22.8"], ["12/15/2022 20:00", "22.9"], ["12/15/2022 20:30", "22.8"], ["12/15/2022 21:00", "22.7"], ["12/15/2022 21:30", "22.7"], ["12/15/2022 22:00", "22.8"], ["12/15/2022 22:30", "22.7"], ["12/15/2022 23:00", "22.8"], ["12/15/2022 23:30", "22.7"], ["12/16/2022 00:00", "22.7"], ["12/16/2022 00:30", "22.7"], ["12/16/2022 01:00", "22.8"], ["12/16/2022 01:30", "22.7"], ["12/16/2022 02:00", "22.7"], ["12/16/2022 02:30", "22.7"], ["12/16/2022 03:00", "22.6"], ["12/16/2022 03:30", "22.7"], ["12/16/2022 04:00", "22.7"], ["12/16/2022 04:30", "22.7"], ["12/16/2022 05:00", "22.7"], ["12/16/2022 05:30", "22.7"], ["12/16/2022 06:00", "22.7"], ["12/16/2022 06:30", "22.6"], ["12/16/2022 07:00", "22.6"], ["12/16/2022 07:30", "22.6"], ["12/16/2022 08:00", "22.7"], ["12/16/2022 08:30", "22.6"], ["12/16/2022 09:00", "22.7"], ["12/16/2022 09:30", "22.6"], ["12/16/2022 10:00", "22.7"], ["12/16/2022 10:30", "22.8"], ["12/16/2022 11:00", "22.8"], ["12/16/2022 11:30", "22.7"], ["12/16/2022 12:00", "22.8"], ["12/16/2022 12:30", "22.9"], ["12/16/2022 13:00", "22.9"], ["12/16/2022 13:30", "22.9"], ["12/16/2022 14:00", "22.9"], ["12/16/2022 14:30", "22.9"], ["12/16/2022 15:00", "22.9"], ["12/16/2022 15:30", "22.9"], ["12/16/2022 16:00", "22.9"], ["12/16/2022 16:30", "22.9"], ["12/16/2022 17:00", "22.9"], ["12/16/2022 17:30", "22.8"], ["12/16/2022 18:00", "22.9"], ["12/16/2022 18:30", "22.8"], ["12/16/2022 19:00", "22.8"], ["12/16/2022 19:30", "22.8"], ["12/16/2022 20:00", "22.8"], ["12/16/2022 20:30", "22.7"], ["12/16/2022 21:00", "22.7"], ["12/16/2022 21:30", "22.7"], ["12/16/2022 22:00", "22.7"], ["12/16/2022 22:30", "22.7"], ["12/16/2022 23:00", "22.7"], ["12/16/2022 23:30", "22.7"], ["12/17/2022 00:00", "22.7"], ["12/17/2022 00:30", "22.7"], ["12/17/2022 01:00", "22.7"], ["12/17/2022 01:30", "22.7"], ["12/17/2022 02:00", "22.7"], ["12/17/2022 02:30", "22.7"], ["12/17/2022 03:00", "22.7"], ["12/17/2022 03:30", "22.5"], ["12/17/2022 04:00", "22.5"], ["12/17/2022 04:30", "22.6"], ["12/17/2022 05:00", "22.6"], ["12/17/2022 05:30", "22.7"], ["12/17/2022 06:00", "22.6"], ["12/17/2022 06:30", "22.4"], ["12/17/2022 07:00", "22.5"], ["12/17/2022 07:30", "22.4"], ["12/17/2022 08:00", "22.4"], ["12/17/2022 08:30", "22.4"], ["12/17/2022 09:00", "22.4"], ["12/17/2022 09:30", "22.4"], ["12/17/2022 10:00", "22.7"], ["12/17/2022 10:30", "22.7"], ["12/17/2022 11:00", "22.6"], ["12/17/2022 11:30", "22.5"], ["12/17/2022 12:00", "22.6"], ["12/17/2022 12:30", "22.5"], ["12/17/2022 13:00", "22.9"], ["12/17/2022 13:30", "22.9"], ["12/17/2022 14:00", "23.1"], ["12/17/2022 14:30", "23.2"], ["12/17/2022 15:00", "23.2"], ["12/17/2022 15:30", "23.2"], ["12/17/2022 16:00", "23.3"], ["12/17/2022 16:30", "23.3"], ["12/17/2022 17:00", "23.4"], ["12/17/2022 17:30", "23.3"], ["12/17/2022 18:00", "23.4"], ["12/17/2022 18:30", "23.4"], ["12/17/2022 19:00", "23.4"], ["12/17/2022 19:30", "23.3"], ["12/17/2022 20:00", "23.5"], ["12/17/2022 20:30", "23.5"], ["12/17/2022 21:00", "23.3"], ["12/17/2022 21:30", "23.4"], ["12/17/2022 22:00", "23.3"], ["12/17/2022 22:30", "23.1"], ["12/17/2022 23:00", "23.3"], ["12/17/2022 23:30", "23.4"], ["12/18/2022 00:00", "23.5"], ["12/18/2022 00:30", "23.5"], ["12/18/2022 01:00", "23.4"], ["12/18/2022 01:30", "23.5"], ["12/18/2022 02:00", "23.6"], ["12/18/2022 02:30", "23.8"], ["12/18/2022 03:00", "23.9"], ["12/18/2022 03:30", "24.1"], ["12/18/2022 04:00", "24"], ["12/18/2022 04:30", "24.1"], ["12/18/2022 05:00", "24.1"], ["12/18/2022 05:30", "24.1"], ["12/18/2022 06:00", "24"], ["12/18/2022 06:30", "24.1"], ["12/18/2022 07:00", "24.1"], ["12/18/2022 07:30", "24.1"], ["12/18/2022 08:00", "24"], ["12/18/2022 08:30", "23.9"], ["12/18/2022 09:00", "23.9"], ["12/18/2022 09:30", "23.9"], ["12/18/2022 10:00", "24"], ["12/18/2022 10:30", "24"], ["12/18/2022 11:00", "23.9"], ["12/18/2022 11:30", "24"], ["12/18/2022 12:00", "24"], ["12/18/2022 12:30", "24"], ["12/18/2022 13:00", "24"], ["12/18/2022 13:30", "24"], ["12/18/2022 14:00", "24"], ["12/18/2022 14:30", "23.9"], ["12/18/2022 15:00", "23.9"], ["12/18/2022 15:30", "23.9"], ["12/18/2022 16:00", "24"], ["12/18/2022 16:30", "23.9"], ["12/18/2022 17:00", "23.9"], ["12/18/2022 17:30", "23.7"], ["12/18/2022 18:00", "23.7"], ["12/18/2022 18:30", "23.7"], ["12/18/2022 19:00", "23.7"], ["12/18/2022 19:30", "23.7"], ["12/18/2022 20:00", "23.7"], ["12/18/2022 20:30", "23.7"], ["12/18/2022 21:00", "23.7"], ["12/18/2022 21:30", "23.7"], ["12/18/2022 22:00", "23.5"], ["12/18/2022 22:30", "23.6"], ["12/18/2022 23:00", "23.5"], ["12/18/2022 23:30", "23.5"], ["12/19/2022 00:00", "23.5"], ["12/19/2022 00:30", "23.6"], ["12/19/2022 01:00", "23.5"], ["12/19/2022 01:30", "23.5"], ["12/19/2022 02:00", "23.5"], ["12/19/2022 02:30", "23.5"], ["12/19/2022 03:00", "23.5"], ["12/19/2022 03:30", "23.5"], ["12/19/2022 04:00", "23.5"], ["12/19/2022 04:30", "23.4"], ["12/19/2022 05:00", "23.4"], ["12/19/2022 05:30", "23.3"], ["12/19/2022 06:00", "23.4"], ["12/19/2022 06:30", "23.4"], ["12/19/2022 07:00", "23.3"], ["12/19/2022 07:30", "23.3"], ["12/19/2022 08:00", "23.3"], ["12/19/2022 08:30", "23.3"], ["12/19/2022 09:00", "23.5"], ["12/19/2022 09:30", "23.5"], ["12/19/2022 10:00", "23.5"], ["12/19/2022 10:30", "23.5"], ["12/19/2022 11:00", "23.5"], ["12/19/2022 11:30", "23.5"], ["12/19/2022 12:00", "23.5"], ["12/19/2022 12:30", "23.5"], ["12/19/2022 13:00", "23.5"], ["12/19/2022 13:30", "23.5"], ["12/19/2022 14:00", "23.5"], ["12/19/2022 14:30", "23.6"], ["12/19/2022 15:00", "23.6"], ["12/19/2022 15:30", "23.5"], ["12/19/2022 16:00", "23.5"], ["12/19/2022 16:30", "23.6"], ["12/19/2022 17:00", "23.6"], ["12/19/2022 17:30", "23.5"], ["12/19/2022 18:00", "23.6"], ["12/19/2022 18:30", "23.5"], ["12/19/2022 19:00", "23.5"], ["12/19/2022 19:30", "23.5"], ["12/19/2022 20:00", "23.4"], ["12/19/2022 20:30", "23.4"], ["12/19/2022 21:00", "23.3"], ["12/19/2022 21:30", "23.4"], ["12/19/2022 22:00", "23.3"], ["12/19/2022 22:30", "23.3"], ["12/19/2022 23:00", "23.3"], ["12/19/2022 23:30", "23.2"], ["12/20/2022 00:00", "23.2"], ["12/20/2022 00:30", "23.1"], ["12/20/2022 01:00", "23.2"], ["12/20/2022 01:30", "23.2"], ["12/20/2022 02:00", "22.9"], ["12/20/2022 02:30", "23.1"], ["12/20/2022 03:00", "23"], ["12/20/2022 03:30", "23.1"], ["12/20/2022 04:00", "22.9"], ["12/20/2022 04:30", "23"], ["12/20/2022 05:00", "22.9"], ["12/20/2022 05:30", "22.9"], ["12/20/2022 06:00", "22.9"], ["12/20/2022 06:30", "22.9"], ["12/20/2022 07:00", "22.9"], ["12/20/2022 07:30", "22.8"], ["12/20/2022 08:00", "22.8"], ["12/20/2022 08:30", "22.9"], ["12/20/2022 09:00", "22.9"], ["12/20/2022 09:30", "22.9"], ["12/20/2022 10:00", "23.7"], ["12/20/2022 10:30", "27.1"], ["12/20/2022 11:00", "28.6"], ["12/20/2022 11:30", "29.8"], ["12/20/2022 12:00", "31.3"], ["12/20/2022 12:30", "31.8"], ["12/20/2022 13:00", "32"], ["12/20/2022 13:30", "32.1"], ["12/20/2022 14:00", "32.1"], ["12/20/2022 14:30", "32.1"], ["12/20/2022 15:00", "32"], ["12/20/2022 15:30", "31.8"], ["12/20/2022 16:00", "31.6"], ["12/20/2022 16:30", "31.3"], ["12/20/2022 17:00", "31.1"]]
  in  "範圍":cluster{"Cell1":string, "Cell2":string}={"Cell1"="A1", "Cell2"="B1262"}
  in  "Sheets":i32=1
  in  "Path":path
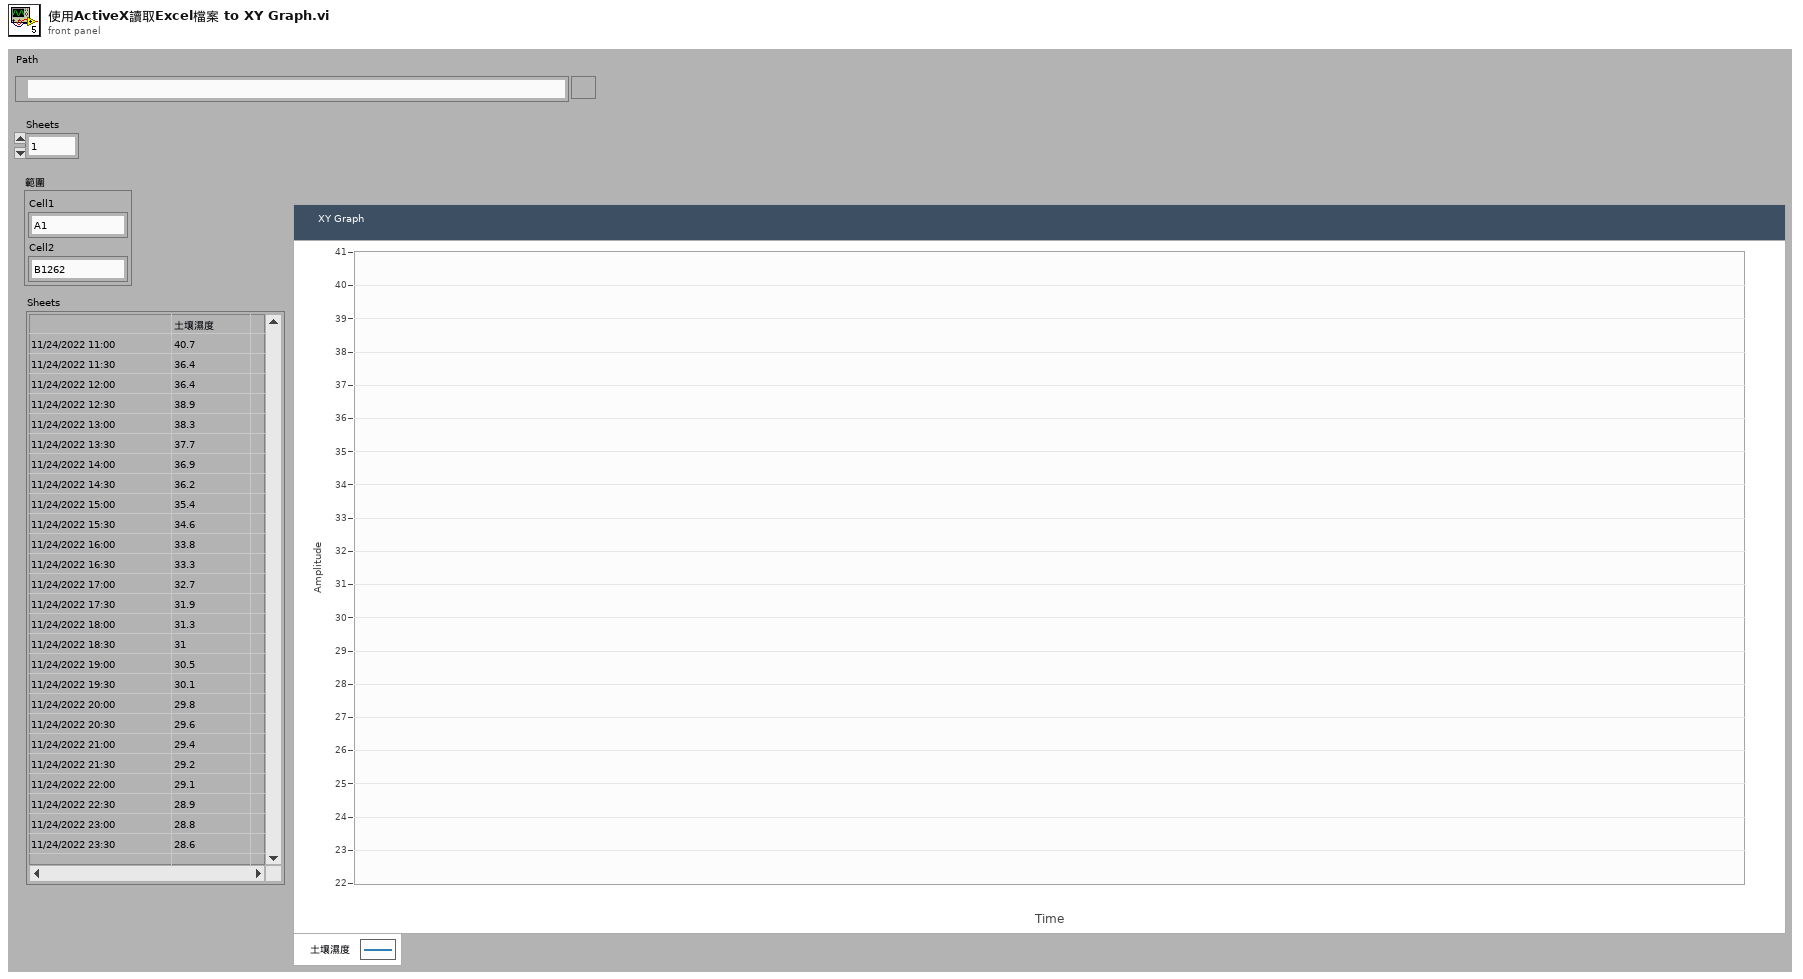
[diagram p1: front panel]
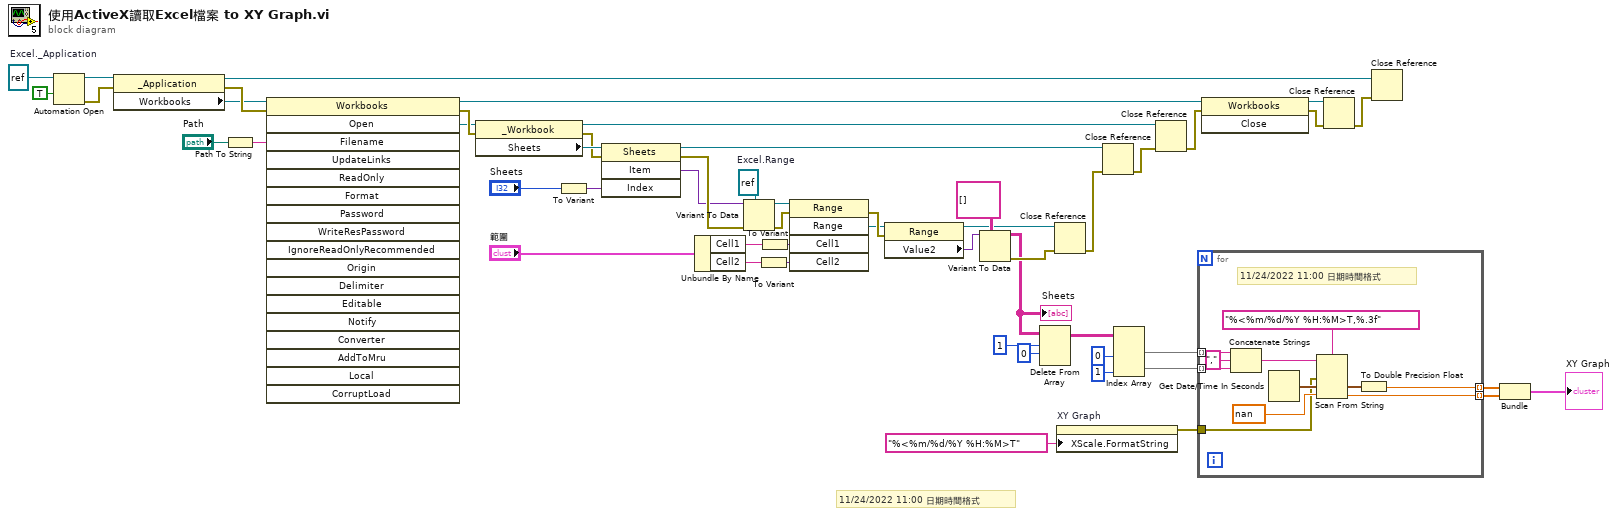
[diagram p0: block diagram]
diagram:
  w40 = refnum<k7> refnum  # Excel.Range
  w47 = refnum<k7> refnum  # Excel._Application
  # "11/24/2022 11:00 日期時間格式"
  n1 = Automation Open(Automation Refnum=w47, 9:TRUE) -> (Automation Refnum=w44:refnum<k7>, error out=w46:errorcluster)  [unwired: 2 in]
  n2 = property class="_Application"(reference=w44, error in=w46) -> (reference out=w30:refnum<k7>, error out=w45:errorcluster, "Workbooks"=w42:refnum<k7>)
  n3 = Path To String(path="Path") -> (string=w52:string)
  n4 = invoke class="Workbooks" method="Open"(reference=w42, error in=w45, "Filename"=w52) -> (reference out=w37:refnum<k7>, error out=w51:errorcluster, "Open"=w41:refnum<k7>)  [unwired: 15 in, 15 out]
  n5 = property class="_Workbook"(reference=w41, error in=w51) -> (reference out=w33:refnum<k7>, error out=w49:errorcluster, "Sheets"=w50:refnum<k7>)
  n6 = To Variant(anything="Sheets") -> (Variant=w38:variant)
  n7 = invoke class="Sheets" method="Item"(reference=w50, error in=w49, "Index"=w38) -> (reference out=w32:refnum<k7>, error out=w48:errorcluster, "Item"=w28:variant)  [unwired: 1 in, 1 out]
  n8 = Unbundle By Name("範圍") -> ("Cell1"=w17:string, "Cell2"=w16:string)
  n9 = Variant To Data(error in=w48, type=w40, Variant=w28) -> (data=w20:refnum<k7>, error out=w21:errorcluster)
  n10 = To Variant(anything=w16) -> (Variant=w25:variant)
  n11 = To Variant(anything=w17) -> (Variant=w26:variant)
  n12 = invoke class="Range" method="Range"(reference=w20, error in=w21, "Cell1"=w26, "Cell2"=w25) -> (error out=w24:errorcluster, "Range"=w23:refnum<k7>)  [unwired: 1 in, 3 out]
  n13 = property class="Range"(reference=w23, error in=w24) -> (reference out=w15:refnum<k7>, "Value2"=w22:variant)  [unwired: 1 out]
  n14 = Variant To Data(type=string[][] [] ("data"), Variant=w22) -> (data=w6:string[][], error out=w14:errorcluster)  [unwired: 1 in]
  "Sheets" <- w6
  n15 = Delete From Array(array=w6, length=1, index (row)=0) -> (array with subset deleted=w5:string[][])  [unwired: 1 in, 1 out]
  n16 = Close Reference(reference=w15, error in (no error)=w14) -> (error out=w19:errorcluster)
  n17 = property on="XY Graph" class="XYGraph (strict)"("XScale.FormatString"="%<%m/%d/%Y %H:%M>T" ("X Scale.Format String")) -> (error out=w1:errorcluster)  [unwired: 2 in, 1 out]
  n18 = Close Reference(reference=w32, error in (no error)=w19) -> (error out=w31:errorcluster)
  n19 = Index Array(array=w5, index (col) #1=0 ("disabled index (col)"), index (col) #2=1 ("index (col)")) -> (element #1=w11:string[], element #2=w10:string[])  [unwired: 2 in]
  n20 = Close Reference(reference=w33, error in (no error)=w31) -> (error out=w36:errorcluster)
  n21 = for {
    tunnel: w11 -> [w63] mode=indexing
    tunnel: w10 -> [w61] mode=indexing
    tunnel: [w57] -> w9 mode=indexing
    tunnel: [w56] -> w8 mode=indexing
    tunnel: w1 -> [w54]
    # "11/24/2022 11:00 日期時間格式"
    n22 = Concatenate Strings(w63, ",", w61) -> (w62:string)
    n23 = Get Date/Time In Seconds() -> (seconds since 1Jan1904=w59:timestamp)
    n24 = Scan From String(format string="%<%m/%d/%Y %H:%M>T,%.3f", input string=w62, error in=w54, default 1=w59, default 2=nan ("default value 2")) -> (output 1=w58:timestamp, output 2=w56:dbl)  [unwired: 1 in, 3 out]
    n25 = To Double Precision Float(number=w58) -> (double precision float=w57:dbl)
  }
  n26 = invoke class="Workbooks" method="Close"(reference=w37, error in=w36) -> (reference out=w35:refnum<k7>, error out=w34:errorcluster)  [unwired: 1 in, 1 out]
  n27 = Close Reference(reference=w35, error in (no error)=w34) -> (error out=w29:errorcluster)
  n28 = Close Reference(reference=w30, error in (no error)=w29) -> ()  [unwired: 1 out]
  n29 = Bundle(w9, w8) -> (→"XY Graph":cluster{dbl[], dbl[]})  [unwired: 1 in]
